vi "NISE.remote.Write ActivePhysChan.vi"(8 "error in (no error)":errorcluster, 10 "ActivePhysChan":refnum<k21>, 11 "SLSC Remote in":refnum<class "SLSC Interface.lvclass">) -> (0 "error out":errorcluster, 3 "SLSC Remote out":refnum<class "SLSC Interface.lvclass">)   [LabVIEW 2016, in "SLSC Interface.lvclass"]
uses:
  SLSC Interface Class/SLSC Interface.lvclass
  <vilib>/NI/JSON Support for LabVIEW/JSON Value/JSON Value.lvclass
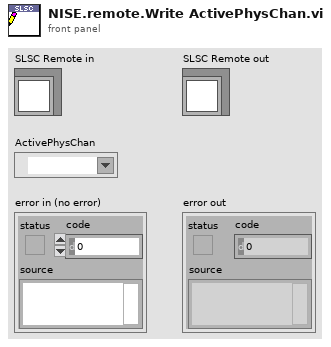
[diagram p1: front panel]
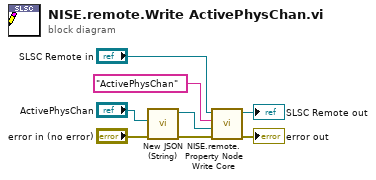
[diagram p0: block diagram]
diagram:
  n1 = call <vilib>:"New JSON (String).vi"("error in (no error)"="error in (no error)", "value"="ActivePhysChan") -> ("error out"=w1:errorcluster, "JSON Value out"=w3:refnum<class "JSON Value.lvclass">)  [unwired: 8 in]
  n2 = call "NISE.remote.Property Node Write Core.vi"("error in (no error)"=w1, "JSON Value in"=w3, "property"="ActivePhysChan", "SLSC Remote in"="SLSC Remote in") -> ("error out"=→"error out":errorcluster, "SLSC Remote out"=→"SLSC Remote out":refnum<class "SLSC Interface.lvclass">)  [unwired: 6 in]
